vi "Pre Launch Init.vi"(11 "CS++OPCUAInterface in":refnum<class "CS++OPCUAInterface.lvclass">) -> (0 "Error Out":errorcluster, 3 "CS++OPCUAInterface out":refnum<class "CS++OPCUAInterface.lvclass">)   [LabVIEW 2015, in "CS++OPCUAInterface.lvlib" / "CS++OPCUAInterface.lvclass"]
doc: "(<B>Filename</B>: Actor Framework.lvlib:Actor.lvclass:Pre Launch Init.vi)\n\nDefines behavior that occurs after the Launch Actor method is invoked but before the actor's Actor Core method begins running.\n\nThe Pre Launch Init method is guaranteed to finish before the Launch Actor method returns to its caller and before the actor itself receives any messages. Any references that the Pre Launch Init method obtains are guaranteed to have the same lifetime as the actor itself. Any errors that the Pre Launch Init method returns will abort the launch.\n\nBy default, this method does nothing. A descendant class may override it to define behavior."
uses:
  CS++OPCUAInterface.lvclass
  CS++OPCUAInterface.lvclass/CS++OPCUAInterface.ctl
  CSPP_Core/Classes/CS++ProcessVariables/ProcessVariable/PV.lvclass
  CSPP_Core/Classes/CS++ProcessVariables/ProcessVariable/PV.lvclass/PV.ctl
  CSPP_Core/Classes/CS++ProcessVariables/ProcessVariable/Write Type Descriptor.vi
  CSPP_Core/Classes/CS++ProcessVariables/ProcessVariable/Write Name.vi
  CSPP_Core/Classes/CS++ProcessVariables/ProcessVariable/Write PV URL.vi
  <vilib>/Utility/error.llb/Error Cluster From Error Code.vi
  CSPP_Core/Actors/CS++BaseActor/CS++BaseActor.lvclass
  <vilib>/OPCUA/NI OPC UA Client.lvlib
  CSPP_Core/Classes/CS++ProcessVariables/CS++ProcessVariables.lvlib
  CSPP_Core/Classes/CS++ProcessVariables/PVConnection/PVConnection.lvclass
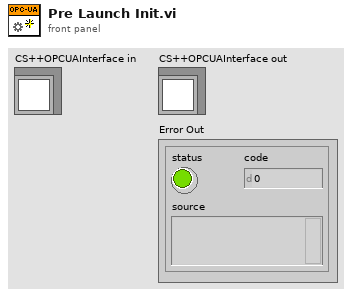
[diagram p1: front panel]
types:
  T1 = cluster{"Read Access":enum8{"Allowed", "Required", "None"}, "Write Access":enum8{"Allowed", "Required", "None"}}
  T2 = cluster{"name":string, "node type":enum32{"Other", "Folder", "Item/Property"}, "DataType":u32, "access":enum16{"Null", "Read", "Write", "Read&Write"}, "description":string}
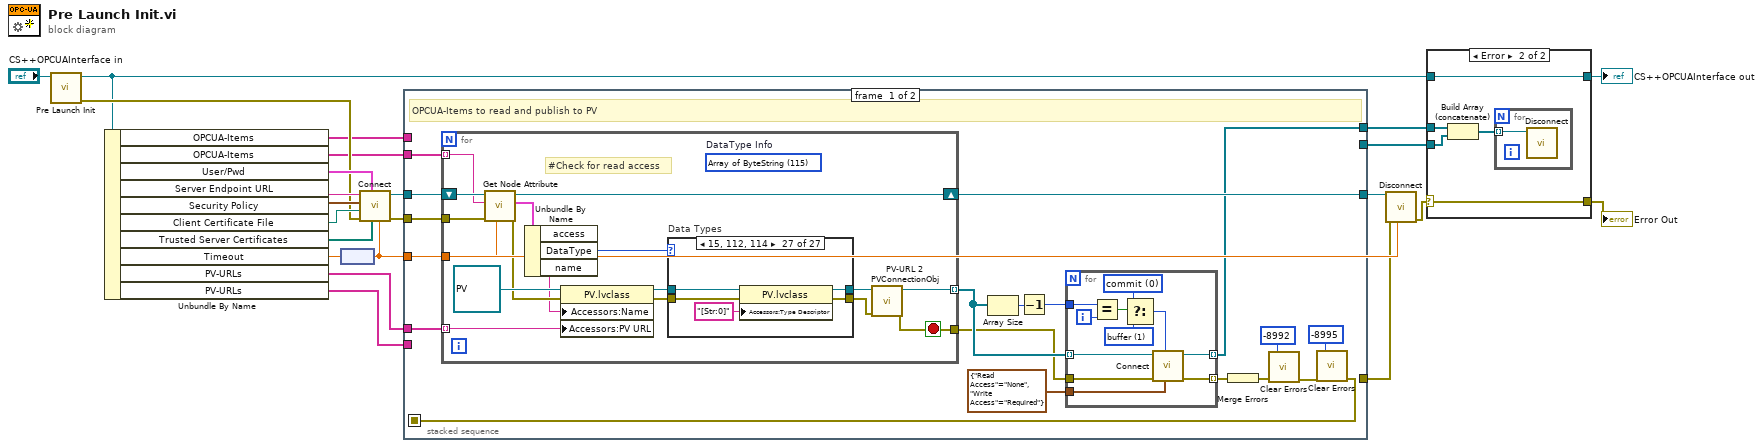
[diagram p0: block diagram]
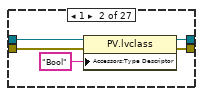
[diagram p3: hidden frame]
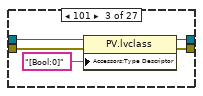
[diagram p4: hidden frame]
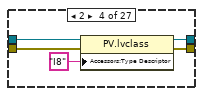
[diagram p5: hidden frame]
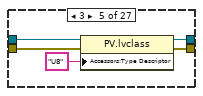
[diagram p6: hidden frame]
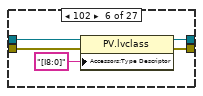
[diagram p7: hidden frame]
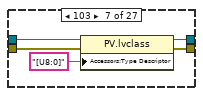
[diagram p8: hidden frame]
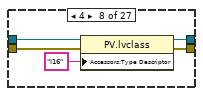
[diagram p9: hidden frame]
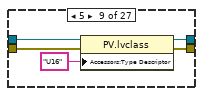
[diagram p10: hidden frame]
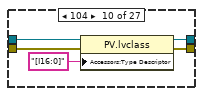
[diagram p11: hidden frame]
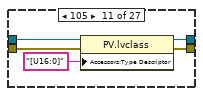
[diagram p12: hidden frame]
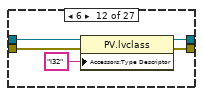
[diagram p13: hidden frame]
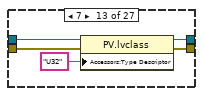
[diagram p14: hidden frame]
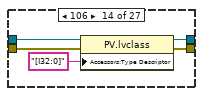
[diagram p15: hidden frame]
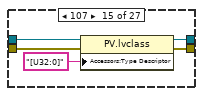
[diagram p16: hidden frame]
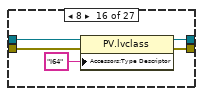
[diagram p17: hidden frame]
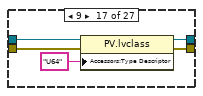
[diagram p18: hidden frame]
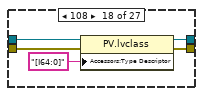
[diagram p19: hidden frame]
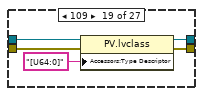
[diagram p20: hidden frame]
diagram:
  n1 = call-parent "Pre Launch Init.vi"("CS++BaseActor in"="CS++OPCUAInterface in") -> ("error out"=w16:errorcluster, "CS++BaseActor out"=w8:refnum<class "CS++OPCUAInterface.lvclass">)  [unwired: 9 in]
  n2 = Unbundle By Name(w8) -> ("OPCUA-Items"=w2:string[], "OPCUA-Items"=w13:string[], "User/Pwd"=w21:cluster{"Username":string, "Password":string}, "Server Endpoint URL"=w22:string, "Security Policy"=w20:cluster{"Message Mode":u16, "Security":u16}, "Client Certificate File"=w19:path, "Trusted Server Certificates"=w18:path[], "Timeout"=w17:dbl[unit], "PV-URLs"=w10:string[], "PV-URLs"=w1:string[])
  n3 = node(w17) -> (w11:dbl)
  n4 = call <vilib>:"Connect.vi"("timeout (5000 ms)"=w11, "trusted server certificates"=w18, "username/password"=w21, "error in (no error)"=w16, "client certificate file"=w19, "security policy"=w20, "server endpoint URL"=w22) -> ("error out"=w14:errorcluster, "OPC UA client refnum out"=w15:refnum<k21>)  [unwired: 2 in, 1 out]
  n5 = stacked-sequence {
    seq-local: [w24 _] -> [_ w203]
    tunnel: w15 -> [w41 w218]
    tunnel: w14 -> [w40 _]
    tunnel: w13 -> [w39 _]
    tunnel: [w38 _] -> w12
    tunnel: w11 -> [w37 w217]
    tunnel: w10 -> [w36 _]
    tunnel: [_ w204] -> w9
    tunnel: [w25 _] -> w6
    tunnel: [_ w206] -> w3
    tunnel: w2 -> [_ w205]
    tunnel: w1 -> [_ w202]
    frame #0 {
      # "OPCUA-Items to read and publish to PV"
      n6 = for {
        tunnel: w39 -> [w67] mode=indexing
        tunnel: w37 -> [w65]
        shift-right: [w66] -> w38
        shift-left: w41 -> [w69]
        tunnel: w36 -> [w62] mode=indexing
        tunnel: [w54] -> w27 mode=indexing
        tunnel: w40 -> [w68]
        tunnel: [w53] -> w26
        stop <- w53 stop-if-true
        (unwired) u32 115 items=["Boolean"=1, "SByte"=2, "Byte"=3, "Int16"=4, "UInt16"=5, "Int32"=6, "UInt32"=7, "Int64"=8, "UInt64"=9, "Float"=10, "Double"=11, "String"=12, "DateTime"=13, "ByteString"=15, "Array of Boolean"=101, "Array of SByte"=102, "Array of Byte"=103, "Array of Int16"=104, "Array of UInt16"=105, "Array of Int32"=106, "Array of UInt32"=107, "Array of Int64"=108, "Array of UInt64"=109, "Array of Float"=110, "Array of Double"=111, "Array of String"=112, "Array of DateTime"=113, "Array of ByteString"=115]  # DataType Info
        # "#Check for read access"
        n7 = call <vilib>:"Get Node Attribute.vi"("timeout (5000 ms)"=w65, "error in (no error)"=w68, "node path"=w67, "OPC UA client refnum in"=w69) -> ("error out"=w63:errorcluster, "node attribute"=w55:T2, "OPC UA client refnum out"=w66:refnum<k21>)  [unwired: 5 in]
        n8 = Unbundle By Name(w55) -> ("DataType"=w58:u32, "name"=w59:string)  [unwired: 1 out]
        n9 = property class="PV.lvclass"(reference=refnum<class "PV.lvclass"> refnum ("CS++ProcessVariables.lvlib:PV.lvclass"), error in=w63, "Accessors:Name"=w59, "Accessors:PV URL"=w62) -> (reference out=w61:refnum<class "PV.lvclass">, error out=w60:errorcluster)
        n10 = case "Data Types" shown="15, 112, 114" w58 {
          tunnel: w61 -> [w71 w76 w81 w86 w91 w96 w101 w106 w111 w116 w121 w126 w131 w136 w141 w146 w151 w156 w161 w166 w171 w176 w181 w186 w191 w196 w201]
          tunnel: w60 -> [w70 w75 w80 w85 w90 w95 w100 w105 w110 w115 w120 w125 w130 w135 w140 w145 w150 w155 w160 w165 w170 w175 w180 w185 w190 w195 w200]
          tunnel: [w71 w74 w79 w84 w89 w94 w99 w104 w109 w114 w119 w124 w129 w134 w139 w144 w149 w154 w159 w164 w169 w174 w179 w184 w189 w194 w199] -> w57
          tunnel: [w70 w73 w78 w83 w88 w93 w98 w103 w108 w113 w118 w123 w128 w133 w138 w143 w148 w153 w158 w163 w168 w173 w178 w183 w188 w193 w198] -> w56
          frame Default {
          }
          frame 1 {
            n11 = property class="PV.lvclass"(reference=w76, error in=w75, "Accessors:Type Descriptor"="Bool" ("Type Descriptor")) -> (reference out=w74:refnum<class "PV.lvclass">, error out=w73:errorcluster)
          }
          frame 101 {
            n12 = property class="PV.lvclass"(reference=w81, error in=w80, "Accessors:Type Descriptor"="[Bool:0]" ("Type Descriptor")) -> (reference out=w79:refnum<class "PV.lvclass">, error out=w78:errorcluster)
          }
          frame 2 {
            n13 = property class="PV.lvclass"(reference=w86, error in=w85, "Accessors:Type Descriptor"="I8" ("Type Descriptor")) -> (reference out=w84:refnum<class "PV.lvclass">, error out=w83:errorcluster)
          }
          frame 3 {
            n14 = property class="PV.lvclass"(reference=w91, error in=w90, "Accessors:Type Descriptor"="U8" ("Type Descriptor")) -> (reference out=w89:refnum<class "PV.lvclass">, error out=w88:errorcluster)
          }
          frame 102 {
            n15 = property class="PV.lvclass"(reference=w96, error in=w95, "Accessors:Type Descriptor"="[I8:0]" ("Type Descriptor")) -> (reference out=w94:refnum<class "PV.lvclass">, error out=w93:errorcluster)
          }
          frame 103 {
            n16 = property class="PV.lvclass"(reference=w101, error in=w100, "Accessors:Type Descriptor"="[U8:0]" ("Type Descriptor")) -> (reference out=w99:refnum<class "PV.lvclass">, error out=w98:errorcluster)
          }
          frame 4 {
            n17 = property class="PV.lvclass"(reference=w106, error in=w105, "Accessors:Type Descriptor"="I16" ("Type Descriptor")) -> (reference out=w104:refnum<class "PV.lvclass">, error out=w103:errorcluster)
          }
          frame 5 {
            n18 = property class="PV.lvclass"(reference=w111, error in=w110, "Accessors:Type Descriptor"="U16" ("Type Descriptor")) -> (reference out=w109:refnum<class "PV.lvclass">, error out=w108:errorcluster)
          }
          frame 104 {
            n19 = property class="PV.lvclass"(reference=w116, error in=w115, "Accessors:Type Descriptor"="[I16:0]" ("Type Descriptor")) -> (reference out=w114:refnum<class "PV.lvclass">, error out=w113:errorcluster)
          }
          frame 105 {
            n20 = property class="PV.lvclass"(reference=w121, error in=w120, "Accessors:Type Descriptor"="[U16:0]" ("Type Descriptor")) -> (reference out=w119:refnum<class "PV.lvclass">, error out=w118:errorcluster)
          }
          frame 6 {
            n21 = property class="PV.lvclass"(reference=w126, error in=w125, "Accessors:Type Descriptor"="I32" ("Type Descriptor")) -> (reference out=w124:refnum<class "PV.lvclass">, error out=w123:errorcluster)
          }
          frame 7 {
            n22 = property class="PV.lvclass"(reference=w131, error in=w130, "Accessors:Type Descriptor"="U32" ("Type Descriptor")) -> (reference out=w129:refnum<class "PV.lvclass">, error out=w128:errorcluster)
          }
          frame 106 {
            n23 = property class="PV.lvclass"(reference=w136, error in=w135, "Accessors:Type Descriptor"="[I32:0]" ("Type Descriptor")) -> (reference out=w134:refnum<class "PV.lvclass">, error out=w133:errorcluster)
          }
          frame 107 {
            n24 = property class="PV.lvclass"(reference=w141, error in=w140, "Accessors:Type Descriptor"="[U32:0]" ("Type Descriptor")) -> (reference out=w139:refnum<class "PV.lvclass">, error out=w138:errorcluster)
          }
          frame 8 {
            n25 = property class="PV.lvclass"(reference=w146, error in=w145, "Accessors:Type Descriptor"="I64" ("Type Descriptor")) -> (reference out=w144:refnum<class "PV.lvclass">, error out=w143:errorcluster)
          }
          frame 9 {
            n26 = property class="PV.lvclass"(reference=w151, error in=w150, "Accessors:Type Descriptor"="U64" ("Type Descriptor")) -> (reference out=w149:refnum<class "PV.lvclass">, error out=w148:errorcluster)
          }
          frame 108 {
            n27 = property class="PV.lvclass"(reference=w156, error in=w155, "Accessors:Type Descriptor"="[I64:0]" ("Type Descriptor")) -> (reference out=w154:refnum<class "PV.lvclass">, error out=w153:errorcluster)
          }
          frame 109 {
            n28 = property class="PV.lvclass"(reference=w161, error in=w160, "Accessors:Type Descriptor"="[U64:0]" ("Type Descriptor")) -> (reference out=w159:refnum<class "PV.lvclass">, error out=w158:errorcluster)
          }
          frame 10 {
            n29 = property class="PV.lvclass"(reference=w166, error in=w165, "Accessors:Type Descriptor"="Sgl" ("Type Descriptor")) -> (reference out=w164:refnum<class "PV.lvclass">, error out=w163:errorcluster)
          }
          frame 110 {
            n30 = property class="PV.lvclass"(reference=w171, error in=w170, "Accessors:Type Descriptor"="[Sgl:0]" ("Type Descriptor")) -> (reference out=w169:refnum<class "PV.lvclass">, error out=w168:errorcluster)
          }
          frame 11 {
            n31 = property class="PV.lvclass"(reference=w176, error in=w175, "Accessors:Type Descriptor"="Dbl" ("Type Descriptor")) -> (reference out=w174:refnum<class "PV.lvclass">, error out=w173:errorcluster)
          }
          frame 13 {
            n32 = property class="PV.lvclass"(reference=w181, error in=w180, "Accessors:Type Descriptor"="T" ("Type Descriptor")) -> (reference out=w179:refnum<class "PV.lvclass">, error out=w178:errorcluster)
          }
          frame 111 {
            n33 = property class="PV.lvclass"(reference=w186, error in=w185, "Accessors:Type Descriptor"="[Dbl:0]" ("Type Descriptor")) -> (reference out=w184:refnum<class "PV.lvclass">, error out=w183:errorcluster)
          }
          frame 113 {
            n34 = property class="PV.lvclass"(reference=w191, error in=w190, "Accessors:Type Descriptor"="[T:0]" ("Type Descriptor")) -> (reference out=w189:refnum<class "PV.lvclass">, error out=w188:errorcluster)
          }
          frame 12 {
            n35 = property class="PV.lvclass"(reference=w196, error in=w195, "Accessors:Type Descriptor"="Str" ("Type Descriptor")) -> (reference out=w194:refnum<class "PV.lvclass">, error out=w193:errorcluster)
          }
          frame 15, 112, 114 {
            n36 = property class="PV.lvclass"(reference=w201, error in=w200, "Accessors:Type Descriptor"="[Str:0]" ("Type Descriptor")) -> (reference out=w199:refnum<class "PV.lvclass">, error out=w198:errorcluster)
          }
        }
        n37 = call "PV-URL 2 PVConnectionObj.vi"("Error In"=w56, "PV"=w57) -> ("Error Out"=w53:errorcluster, "PVConnection"=w54:refnum<class "PVConnection.lvclass">)  [unwired: 7 in, 1 out]
      }
      n38 = Array Size(array=w27) -> (size(s)=w34:i32)
      n39 = Decrement(x=w34) -> (x-1=w35:i32)
      n40 = for {
        tunnel: w27 -> [w52] mode=indexing
        tunnel: [w51] -> w25 mode=indexing
        tunnel: T1 {"Read Access"=enum."None", "Write Access"=enum."Required"} ("Access (R/W allowed)") -> [w50]
        tunnel: [w49] -> w30 mode=indexing
        tunnel: w35 -> [w47]
        tunnel: w26 -> [w42]
        i -> [w48]
        w44 = u16 1 items=["commit", "buffer"] ("Mode (commit)")
        w45 = u16 0 items=["commit", "buffer"] ("Mode (commit)")
        n41 = Equal?(x=w47, y=w48) -> (x = y?=w46:bool)
        n42 = Select(t=w45, s=w46, f=w44) -> (s? t:f=w43:u16)
        n43 = call <vilib>:"Connect.vi"("Access (R/W allowed)"=w50, "Mode (buffer)"=w43, "Error In"=w42, "PVConnection in"=w52) -> ("Error Out"=w49:errorcluster, "PVConnection out"=w51:refnum<class "PVConnection.lvclass">)  [unwired: 6 in]
      }
      n44 = Merge Errors(w30) -> (w32:errorcluster)
      n45 = call <vilib>:"Clear Errors.vi"("error in (no error)"=w32, "specific error code to clear (0: all)"=-8992) -> ("error out"=w33:errorcluster)  [unwired: 4 in, 1 out]
      n46 = call <vilib>:"Clear Errors.vi"("error in (no error)"=w33, "specific error code to clear (0: all)"=-8995) -> ("error out"=w24:errorcluster)  [unwired: 4 in, 1 out]
    }
    frame #1 {
      # "PV to read and write to OPCUA"
      n47 = for {
        tunnel: w205 -> [w244] mode=indexing
        tunnel: w217 -> [w242]
        shift-right: [w243] -> _
        shift-left: w218 -> [w246]
        tunnel: w202 -> [w239] mode=indexing
        tunnel: [w231] -> w208 mode=indexing
        tunnel: w203 -> [w245]
        tunnel: [w230] -> w207
        stop <- w230 stop-if-true
        (unwired) u32 112 items=["Boolean"=1, "SByte"=2, "Byte"=3, "Int16"=4, "UInt16"=5, "Int32"=6, "UInt32"=7, "Int64"=8, "UInt64"=9, "Float"=10, "Double"=11, "String"=12, "DateTime"=13, "ByteString"=15, "Array of Boolean"=101, "Array of SByte"=102, "Array of Byte"=103, "Array of Int16"=104, "Array of UInt16"=105, "Array of Int32"=106, "Array of UInt32"=107, "Array of Int64"=108, "Array of UInt64"=109, "Array of Float"=110, "Array of Double"=111, "Array of String"=112, "Array of DateTime"=113, "Array of ByteString"=115]  # DataType Info
        # "#Check for write access"
        n48 = call <vilib>:"Get Node Attribute.vi"("timeout (5000 ms)"=w242, "error in (no error)"=w245, "node path"=w244, "OPC UA client refnum in"=w246) -> ("error out"=w240:errorcluster, "node attribute"=w232:T2, "OPC UA client refnum out"=w243:refnum<k21>)  [unwired: 5 in]
        n49 = Unbundle By Name(w232) -> ("DataType"=w235:u32, "name"=w236:string)  [unwired: 1 out]
        n50 = property class="PV.lvclass"(reference=refnum<class "PV.lvclass"> refnum ("CS++ProcessVariables.lvlib:PV.lvclass"), error in=w240, "Accessors:Name"=w236, "Accessors:PV URL"=w239) -> (reference out=w238:refnum<class "PV.lvclass">, error out=w237:errorcluster)
        n51 = case "Data Types" shown="106, 107" w235 {
          tunnel: w238 -> [w248 w253 w258 w263 w268 w273 w278 w283 w288 w293 w298 w303 w308 w313 w318 w323 w328]
          tunnel: w237 -> [w247 w252 w257 w262 w267 w272 w277 w282 w287 w292 w297 w302 w307 w312 w317 w322 w327]
          tunnel: [w248 w251 w256 w261 w266 w271 w276 w281 w286 w291 w296 w301 w306 w311 w316 w321 w326] -> w234
          tunnel: [w247 w250 w255 w260 w265 w270 w275 w280 w285 w290 w295 w300 w305 w310 w315 w320 w325] -> w233
          frame Default {
          }
          frame 1 {
            n52 = property class="PV.lvclass"(reference=w253, error in=w252, "Accessors:Type Descriptor"="B:1" ("Type Descriptor")) -> (reference out=w251:refnum<class "PV.lvclass">, error out=w250:errorcluster)
          }
          frame 101 {
            n53 = property class="PV.lvclass"(reference=w258, error in=w257, "Accessors:Type Descriptor"="B:N" ("Type Descriptor")) -> (reference out=w256:refnum<class "PV.lvclass">, error out=w255:errorcluster)
          }
          frame 2, 3 {
            n54 = property class="PV.lvclass"(reference=w263, error in=w262, "Accessors:Type Descriptor"="C:1" ("Type Descriptor")) -> (reference out=w261:refnum<class "PV.lvclass">, error out=w260:errorcluster)
          }
          frame 102, 103 {
            n55 = property class="PV.lvclass"(reference=w268, error in=w267, "Accessors:Type Descriptor"="C:N" ("Type Descriptor")) -> (reference out=w266:refnum<class "PV.lvclass">, error out=w265:errorcluster)
          }
          frame 4, 5 {
            n56 = property class="PV.lvclass"(reference=w273, error in=w272, "Accessors:Type Descriptor"="S:1" ("Type Descriptor")) -> (reference out=w271:refnum<class "PV.lvclass">, error out=w270:errorcluster)
          }
          frame 104, 105 {
            n57 = property class="PV.lvclass"(reference=w278, error in=w277, "Accessors:Type Descriptor"="S:N" ("Type Descriptor")) -> (reference out=w276:refnum<class "PV.lvclass">, error out=w275:errorcluster)
          }
          frame 6, 7 {
            n58 = property class="PV.lvclass"(reference=w283, error in=w282, "Accessors:Type Descriptor"="I:1" ("Type Descriptor")) -> (reference out=w281:refnum<class "PV.lvclass">, error out=w280:errorcluster)
          }
          frame 106, 107 {
            n59 = property class="PV.lvclass"(reference=w288, error in=w287, "Accessors:Type Descriptor"="I:N" ("Type Descriptor")) -> (reference out=w286:refnum<class "PV.lvclass">, error out=w285:errorcluster)
          }
          frame 8, 9 {
            n60 = property class="PV.lvclass"(reference=w293, error in=w292, "Accessors:Type Descriptor"="L:1" ("Type Descriptor")) -> (reference out=w291:refnum<class "PV.lvclass">, error out=w290:errorcluster)
          }
          frame 108, 109 {
            n61 = property class="PV.lvclass"(reference=w298, error in=w297, "Accessors:Type Descriptor"="L:N" ("Type Descriptor")) -> (reference out=w296:refnum<class "PV.lvclass">, error out=w295:errorcluster)
          }
          frame 10 {
            n62 = property class="PV.lvclass"(reference=w303, error in=w302, "Accessors:Type Descriptor"="F:1" ("Type Descriptor")) -> (reference out=w301:refnum<class "PV.lvclass">, error out=w300:errorcluster)
          }
          frame 110 {
            n63 = property class="PV.lvclass"(reference=w308, error in=w307, "Accessors:Type Descriptor"="F:N" ("Type Descriptor")) -> (reference out=w306:refnum<class "PV.lvclass">, error out=w305:errorcluster)
          }
          frame 11, 13 {
            n64 = property class="PV.lvclass"(reference=w313, error in=w312, "Accessors:Type Descriptor"="D:1" ("Type Descriptor")) -> (reference out=w311:refnum<class "PV.lvclass">, error out=w310:errorcluster)
          }
          frame 111, 113 {
            n65 = property class="PV.lvclass"(reference=w318, error in=w317, "Accessors:Type Descriptor"="D:N" ("Type Descriptor")) -> (reference out=w316:refnum<class "PV.lvclass">, error out=w315:errorcluster)
          }
          frame 12 {
            n66 = property class="PV.lvclass"(reference=w323, error in=w322, "Accessors:Type Descriptor"="C:100" ("Type Descriptor")) -> (reference out=w321:refnum<class "PV.lvclass">, error out=w320:errorcluster)
          }
          frame 15, 112, 114 {
            n67 = property class="PV.lvclass"(reference=w328, error in=w327, "Accessors:Type Descriptor"="C" ("Type Descriptor")) -> (reference out=w326:refnum<class "PV.lvclass">, error out=w325:errorcluster)
          }
        }
        n68 = call "PV-URL 2 PVConnectionObj.vi"("Error In"=w233, "PV"=w234) -> ("Error Out"=w230:errorcluster, "PVConnection"=w231:refnum<class "PVConnection.lvclass">)  [unwired: 7 in, 1 out]
      }
      n69 = Array Size(array=w208) -> (size(s)=w215:i32)
      n70 = Decrement(x=w215) -> (x-1=w216:i32)
      n71 = for {
        tunnel: w208 -> [w229] mode=indexing
        tunnel: [w228] -> w206 mode=indexing
        tunnel: T1 {"Read Access"=enum."Required", "Write Access"=enum."None"} ("Access (R/W allowed)") -> [w227]
        tunnel: [w226] -> w211 mode=indexing
        tunnel: w216 -> [w224]
        tunnel: w207 -> [w219]
        i -> [w225]
        w221 = u16 1 items=["commit", "buffer"] ("Mode (commit)")
        w222 = u16 0 items=["commit", "buffer"] ("Mode (commit)")
        n72 = Equal?(x=w224, y=w225) -> (x = y?=w223:bool)
        n73 = Select(t=w222, s=w223, f=w221) -> (s? t:f=w220:u16)
        n74 = call <vilib>:"Connect.vi"("Access (R/W allowed)"=w227, "Mode (buffer)"=w220, "Error In"=w219, "PVConnection in"=w229) -> ("Error Out"=w226:errorcluster, "PVConnection out"=w228:refnum<class "PVConnection.lvclass">)  [unwired: 6 in]
      }
      n75 = Merge Errors(w211) -> (w213:errorcluster)
      n76 = call <vilib>:"Clear Errors.vi"("error in (no error)"=w213, "specific error code to clear (0: all)"=-8992) -> ("error out"=w214:errorcluster)  [unwired: 4 in, 1 out]
      n77 = call <vilib>:"Clear Errors.vi"("error in (no error)"=w214, "specific error code to clear (0: all)"=-8995) -> ("error out"=w204:errorcluster)  [unwired: 4 in, 1 out]
    }
  }
  n78 = call <vilib>:"Disconnect.vi"("timeout (5000 ms)"=w11, "error in (no error)"=w9, "OPC UA client refnum in"=w12) -> ("error out"=w5:errorcluster)  [unwired: 8 in]
  n79 = case shown="Error" w5 {
    selector: w5 -> [w330 w336]
    tunnel: w8 -> [w333 w338]
    tunnel: [w332 w338] -> w7
    tunnel: w6 -> [w331 w337]
    tunnel: [w330 w336] -> w4
    tunnel: w3 -> [w329 w334]
    frame No Error {
      n80 = Bundle By Name(cluster=w333, "PVConnections Write"=w331, "PVConnections Read"=w329) -> (w332:refnum<class "CS++OPCUAInterface.lvclass">)
    }
    frame Error {
      n81 = Build Array (concatenate)(w337, w334) -> (w335:refnum<class "PVConnection.lvclass">[])
      n82 = for {
        tunnel: w335 -> [w339] mode=indexing
        n83 = call <vilib>:"Disconnect.vi"("PVConnection in"=w339) -> ()  [unwired: 9 in, 2 out]
      }
    }
  }
  "Error Out" <- w4
  "CS++OPCUAInterface out" <- w7
